vi "initialise.vi"(8 "error in (no error)":errorcluster, 11 "ImagingModeDL100901FlexTrajectory in":refnum<class "ImagingModeDL100901FlexTrajectory.lvclass">) -> (0 "error out":errorcluster, 3 "ImagingModeDL100901FlexTrajectory out":refnum<class "ImagingModeDL100901FlexTrajectory.lvclass">)   [LabVIEW 2010, in "ImagingModeDL100901FlexTrajectory.lvclass"]
doc: "The dynamic dispatch-version of this VI initalises the plug-in object by allocating and initalising any dynamic resources need."
uses:
  ImagingModeDL100901FlexTrajectory.lvclass
  ImagingModeDL091001Scaffold/ImagingModeDL091001Scaffold/ImagingModeDL091001Scaffold.lvclass
  Instrument/GenericInstrument/GenericInstrument/GenericInstrument.lvclass
  DAQ/GenericDAQ/GenericDAQ/GenericDAQ.lvclass
  Display/GenericDisplay/GenericDisplay/GenericDisplay.lvclass
  Analyser/GenericAnalyser/GenericAnalyser/GenericAnalyser.lvclass
  ScanHead/GenericScanHead/GenericScanHead/GenericScanHead.lvclass
  Stimulator/GenericStimulator/GenericStimulator/GenericStimulator.lvclass
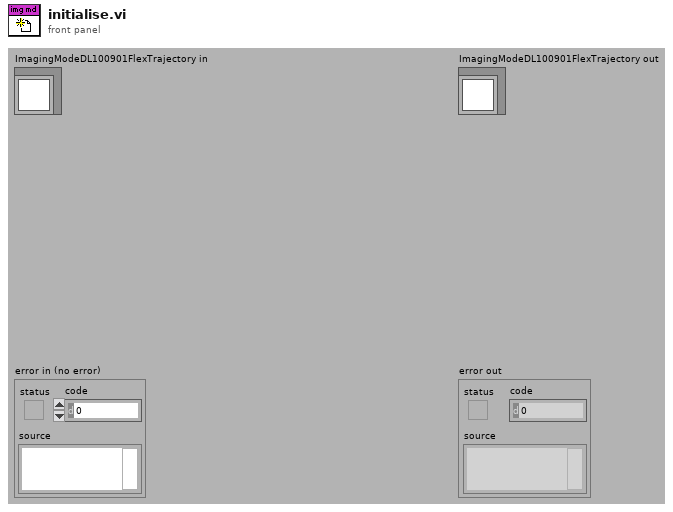
[diagram p1: front panel]
types:
  T1 = typedef "controls_refs.ctl" = cluster{"scan start button":refnum<vi>, "tabs":cluster{"main":refnum<vi>, "settings":refnum<vi>}, "subpanels":cluster{"imagingMode":refnum<vi>, "scanHead":refnum<vi>, "display":refnum<vi>, "experimentController":refnum<vi>, "instrument":refnum<vi>, "stage":refnum<vi>, "stimulator":refnum<vi>, "dataCollection":refnum<vi>, "analyser":refnum<vi>, "daq":refnum<vi>, "imageAssembler":refnum<vi>}, "drop-downs":cluster{"run mode":refnum<vi>, "imagingMode":refnum<vi>, "experimentalController":refnum<vi>, "objective":refnum<vi>}, "status lights":cluster{"experimentController":refnum<vi>, "imagingMode":refnum<vi>, "scanHead":refnum<vi>, "daq":refnum<vi>, "imageAssembler":refnum<vi>, "dataCollection":refnum<vi>, "display":refnum<vi>, "analyser":refnum<vi>, "stage":refnum<vi>, "stimulator":refnum<vi>, "instrument":refnum<vi>}, "message":refnum<vi>, "stimulator enabled?":refnum<vi>, "saving":cluster{"data folder path":refnum<vi>, "file base name":refnum<vi>, "notebook":refnum<vi>}, "progress bar":refnum<vi>, "update icon":refnum<vi>, "title":refnum<vi>, "main vi":refnum<vi>, "user":refnum<vi>, "exit_button":refnum<vi>, "CPU usage %":refnum<vi>}
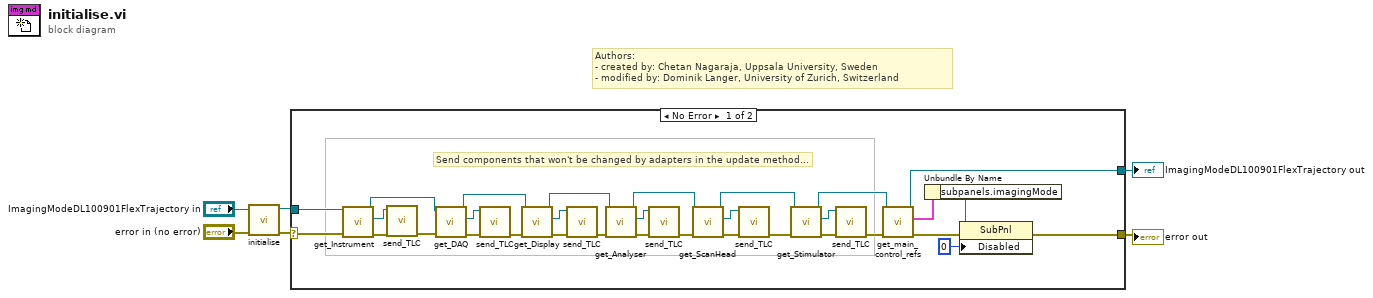
[diagram p0: block diagram]
diagram:
  # "Authors: \n- created by: Chetan Nagaraja, Uppsala University, Sweden\n- modified by: Dominik Langer, University of Zurich, Switzerland"
  n1 = call-parent "initialise.vi"("error in (no error)"="error in (no error)", "GenericPlugin in"="ImagingModeDL100901FlexTrajectory in") -> ("error out"=w2:errorcluster, "GenericPlugin out"=w3:refnum<class "ImagingModeDL100901FlexTrajectory.lvclass">)  [unwired: 8 out]
  n2 = case shown="No Error" w2 {
    selector: w2 -> [w11 w39]
    tunnel: w3 -> [w14 w40]
    tunnel: [w8 w39] -> w1
    tunnel: [w7 w40] -> w4
    frame No Error {
      # "Send components that won't be changed by adapters in the update method..."
      n3 = call-dynamic "get_Instrument.vi"("error in (no error)"=w11, "ScanModeDL090923Scaffold in"=w14) -> ("error out"=w10:errorcluster, "Instrument"=w12:refnum<class "GenericInstrument.lvclass">, "ScanModeDL090923Scaffold out"=w13:refnum<class "ImagingModeDL100901FlexTrajectory.lvclass">)  [unwired: 4 in, 3 out]
      n4 = call-dynamic "send_TLC.vi"("error in (no error)"=w10, "GenericToplevelComponent in"=w12) -> ("error out"=w9:errorcluster)  [unwired: 8 in, 1 out]
      n5 = call-dynamic "get_DAQ.vi"("error in (no error)"=w9, "ScanModeDL090923Scaffold in"=w13) -> ("error out"=w32:errorcluster, "DAQ"=w31:refnum<class "GenericDAQ.lvclass">, "ScanModeDL090923Scaffold out"=w30:refnum<class "ImagingModeDL100901FlexTrajectory.lvclass">)  [unwired: 4 in, 3 out]
      n6 = call-dynamic "send_TLC.vi"("error in (no error)"=w32, "GenericToplevelComponent in"=w31) -> ("error out"=w29:errorcluster)  [unwired: 8 in, 1 out]
      n7 = call-dynamic "get_Display.vi"("error in (no error)"=w29, "ScanModeDL090923Scaffold in"=w30) -> ("error out"=w37:errorcluster, "Display"=w38:refnum<class "GenericDisplay.lvclass">, "ScanModeDL090923Scaffold out"=w27:refnum<class "ImagingModeDL100901FlexTrajectory.lvclass">)  [unwired: 7 out]
      n8 = call-dynamic "send_TLC.vi"("error in (no error)"=w37, "GenericToplevelComponent in"=w38) -> ("error out"=w28:errorcluster)  [unwired: 8 in, 1 out]
      n9 = call-dynamic "get_Analyser.vi"("error in (no error)"=w28, "ScanModeDL090923Scaffold in"=w27) -> ("error out"=w26:errorcluster, "Analyser"=w25:refnum<class "GenericAnalyser.lvclass">, "ScanModeDL090923Scaffold out"=w23:refnum<class "ImagingModeDL100901FlexTrajectory.lvclass">)  [unwired: 4 in, 3 out]
      n10 = call-dynamic "send_TLC.vi"("error in (no error)"=w26, "GenericToplevelComponent in"=w25) -> ("error out"=w24:errorcluster)  [unwired: 8 in, 1 out]
      n11 = call-dynamic "get_ScanHead.vi"("error in (no error)"=w24, "ScanModeDL090923Scaffold in"=w23) -> ("error out"=w20:errorcluster, "ScanHead"=w18:refnum<class "GenericScanHead.lvclass">, "ScanModeDL090923Scaffold out"=w17:refnum<class "ImagingModeDL100901FlexTrajectory.lvclass">)  [unwired: 4 in, 3 out]
      n12 = call-dynamic "send_TLC.vi"("error in (no error)"=w20, "GenericToplevelComponent in"=w18) -> ("error out"=w19:errorcluster)  [unwired: 8 in, 1 out]
      n13 = call-dynamic "get_Stimulator.vi"("error in (no error)"=w19, "ScanModeDL090923Scaffold in"=w17) -> ("error out"=w22:errorcluster, "Stimulator"=w21:refnum<class "GenericStimulator.lvclass">, "ScanModeDL090923Scaffold out"=w15:refnum<class "ImagingModeDL100901FlexTrajectory.lvclass">)  [unwired: 4 in, 3 out]
      n14 = call-dynamic "send_TLC.vi"("error in (no error)"=w22, "GenericToplevelComponent in"=w21) -> ("error out"=w16:errorcluster)  [unwired: 8 in, 1 out]
      n15 = call-dynamic "get_main_control_refs.vi"("error in (no error)"=w16, "GenericPlugin.lvclass in"=w15) -> ("error out"=w35:errorcluster, "control references"=w33:T1, "GenericPlugin.lvclass out"=w7:refnum<class "ImagingModeDL100901FlexTrajectory.lvclass">)  [unwired: 7 out]
      n16 = Unbundle By Name(w33) -> ("subpanels.imagingMode"=w34:refnum<vi>)
      n17 = property class="SubPnl"(reference=w34, error in=w35, "Disabled"=u8 0) -> (error out=w8:errorcluster)  [unwired: 1 out]
    }
    frame Error {
    }
  }
  "error out" <- w1
  "ImagingModeDL100901FlexTrajectory out" <- w4
